vi "GeradorFakeFuncao.vi"() -> ()   [LabVIEW 2018]
uses:
  <vilib>/express/express analysis/Spectral/Block/exnSpectralBlock spectral measurements peak poly.vi
  <vilib>/express/express analysis/Spectral/Block/exnSpectralBlock spectral measurements peak WFM.vi
  <vilib>/express/express analysis/Spectral/XNode/ExpressSpectralMeasurementsBlockNode.xnode
panel:
  out "Waveform Graph":cluster{"f0":dbl, "df":dbl, "magnitude":dbl[]}(graph)
  out "XY Graph 2":cluster{dbl[], dbl[]}(graph)
  out "XY Graph":cluster{dbl[], dbl[]}(graph)
  in  "stop":bool
  in  "Número de Harmônicas":dbl
  in  "Amplitude":dbl
  in  "Frequência":dbl
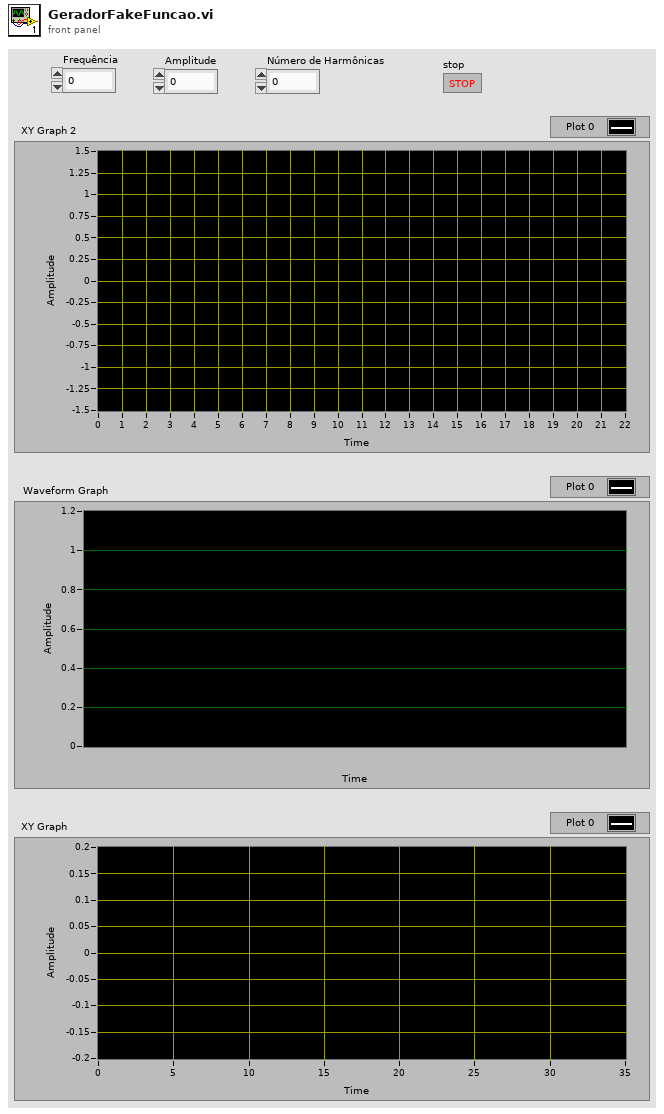
[diagram p1: front panel]
types:
  T1 = cluster{"averaging mode":u16, "weighting mode":u16, "number of averages":u32}
  T2 = cluster{"dB On (F)":bool, "unwrap phase (F)":bool, "convert to degree (F)":bool}
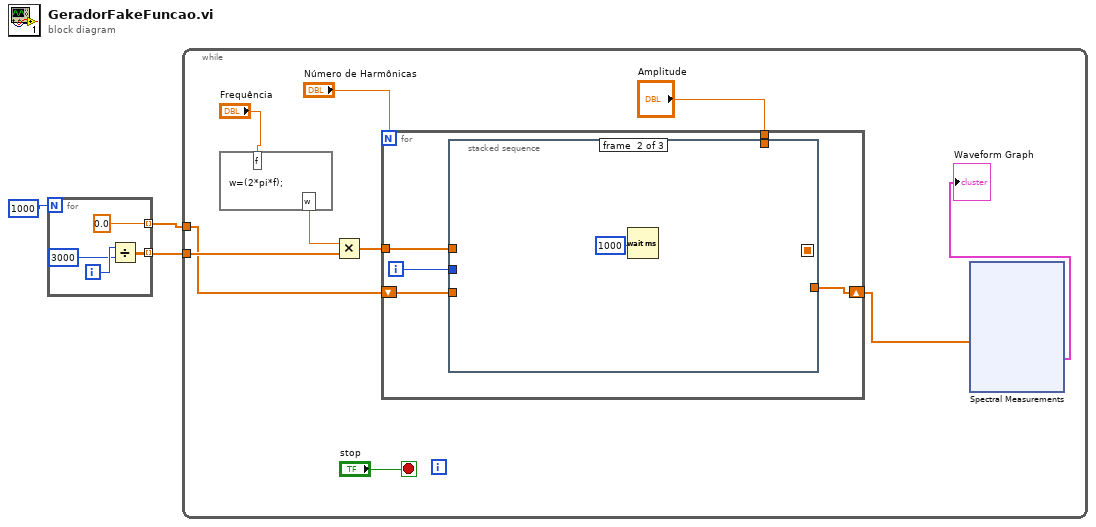
[diagram p0: block diagram]
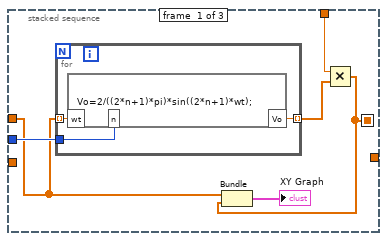
[diagram p2: hidden frame]
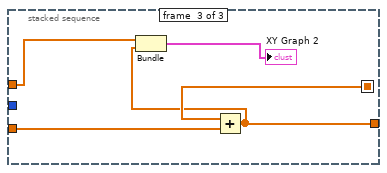
[diagram p3: hidden frame]
diagram:
  n1 = for {
    N: 1000 -> [_]
    tunnel: [w5] -> w2 mode=indexing
    tunnel: [0.0 ("Frequência 2")] -> w1 mode=indexing
    i -> [w7]
    n2 = Divide(x=w7, y=3000) -> (x/y=w5:dbl)
  }
  n3 = while {
    tunnel: w2 -> [w12]
    tunnel: w1 -> [w11]
    stop <- "stop" stop-if-true
    n4 = formula code="w=(2*pi*f);"("f"="Frequência") -> ("w"=w14:dbl)
    n5 = Multiply(x=w14, y=w12) -> (x*y=w15:dbl[])
    n6 = for {
      N: "Número de Harmônicas" -> [_]
      tunnel: w15 -> [w31]
      shift-right: [w29] -> w9
      shift-left: w11 -> [w30]
      tunnel: "Amplitude" -> [w28]
      i -> [w32]
      n7 = stacked-sequence {
        seq-local: [w33 _ _] -> [_ _ w46]
        tunnel: w32 -> [w38 _ _]
        tunnel: w31 -> [w36 _ w45]
        tunnel: w30 -> [_ _ w47]
        tunnel: [_ _ w44] -> w29
        tunnel: w28 -> [w35 _ _]
        frame #0 {
          n8 = for {
            tunnel: w36 -> [w41] mode=indexing
            tunnel: w38 -> [w40]
            tunnel: [w39] -> w34 mode=indexing
            n9 = formula code="Vo=2/((2*n+1)*pi)*sin((2*n+1)*wt);"("wt"=w41, "n"=w40) -> ("Vo"=w39:dbl)
          }
          n10 = Multiply(x=w35, y=w34) -> (x*y=w33:dbl[])
          n11 = Bundle(w36, w33) -> (→"XY Graph":cluster{dbl[], dbl[]})  [unwired: 1 in]
        }
        frame #1 {
          n12 = Wait (ms)(milliseconds to wait=1000) -> ()  [unwired: 1 out]
        }
        frame #2 {
          n13 = Add(x=w46, y=w47) -> (x+y=w44:dbl[])
          n14 = Bundle(w45, w44) -> (→"XY Graph 2":cluster{dbl[], dbl[]})  [unwired: 1 in]
        }
      }
    }
    n15 = xnode "Spectral Measurements"("Signals"=w9) -> ("FFT - (Peak)"=→"Waveform Graph":cluster{"f0":dbl, "df":dbl, "magnitude":dbl[]})  [unwired: 1 in, 2 out]
  }
